vi "Update Tree Parent.vi"(8 "error in":errorcluster, 11 "Report Viewer in":refnum<class "Report Viewer.lvclass">) -> (0 "error out":errorcluster, 2 "Tree Items Parent":string, 3 "Report Viewer out":refnum<class "Report Viewer.lvclass">)   [LabVIEW 2019, in "Report Viewer.lvlib" / "Report Viewer.lvclass"]
uses:
  Library/Report Viewer.lvclass
  Library/Report Viewer.lvclass/Report Viewer.ctl
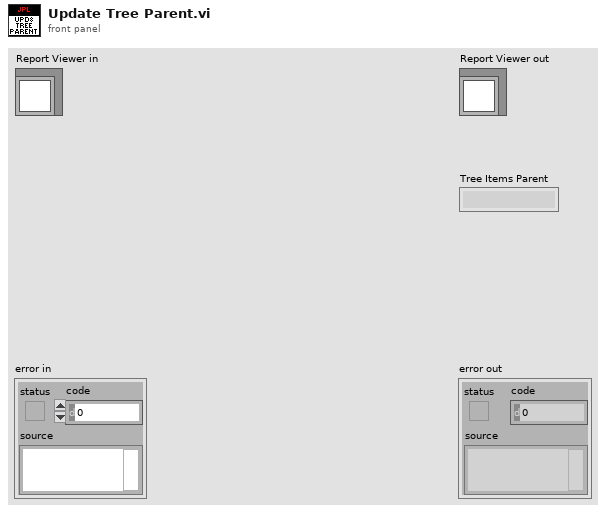
[diagram p1: front panel]
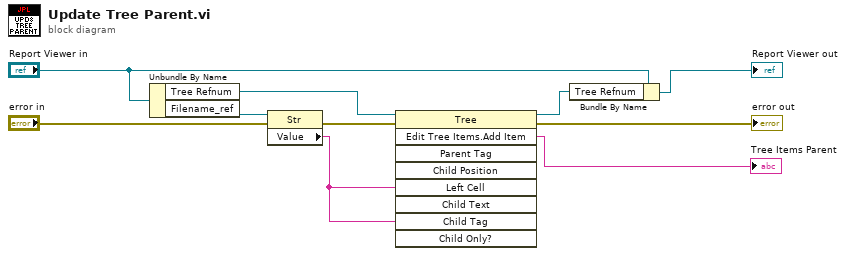
[diagram p0: block diagram]
diagram:
  n1 = Unbundle By Name("Report Viewer in") -> ("Tree Refnum"=w10:refnum<vi>, "Filename_ref"=w8:refnum<vi>)
  n2 = property class="Str"(reference=w8, error in="error in") -> (error out=w9:errorcluster, "Value"=w1:string)  [unwired: 1 out]
  n3 = invoke on="Invoke Node" class="Tree" method="Edit Tree Items.Add Item"(reference=w10, error in=w9, "Left Cell"=w1, "Child Tag"=w1) -> (reference out=w4:refnum<vi>, error out=→"error out":errorcluster, "Edit Tree Items:Add Item"=→"Tree Items Parent":string)  [unwired: 5 in, 6 out]
  n4 = Bundle By Name(cluster="Report Viewer in", "Tree Refnum"=w4) -> (→"Report Viewer out":refnum<class "Report Viewer.lvclass">)
